vi "SRDG535.evt Call Set Trigger.vi"(0 "i ref in":refnum<vi>, 2 "Generator Instance":string="N/A", 3 "Trigger Settings":T1={"trigger"=0, "Impedance"=FALSE, "Slope"=FALSE, "burst count"=2, "external level (V)"=0.0, "Internal/Burst Rate (Hz)"=0.001, "Burst Period"=4} {"Burst Period" min=4 max=32766; "Internal/Burst Rate (Hz)" min=0.001 max=1000000.0 format="%.3f"; "external level (V)" min=-2.56 max=2.56 format="%.2f"; "burst count" min=2 max=32766; "trigger" scale=0.0..4.0}, 5 "error IO":errorcluster) -> (14 "i ref out":refnum<vi>, 19 "error out":errorcluster)   [LabVIEW 2014, in "SRDG535.lvlib"]
doc: "This VI sends a simple event call."
uses:
  SRDG535.lvlib
  SRDG535.Trigger.ctl
  CSCore/CSSystem/CoreLib/CoreLib.double 2 byte array.vi
  CSCore/CSSystem/CoreLib/CoreLib.int 2 byte array.vi
  CSCore/CSSystem/CoreLib/CoreLib.short 2 byte array.vi
  CSCore/CSSystem/CoreLib/CoreLib.lvlib
  CSCore/BaseProcess/BaseProcess.lvlib
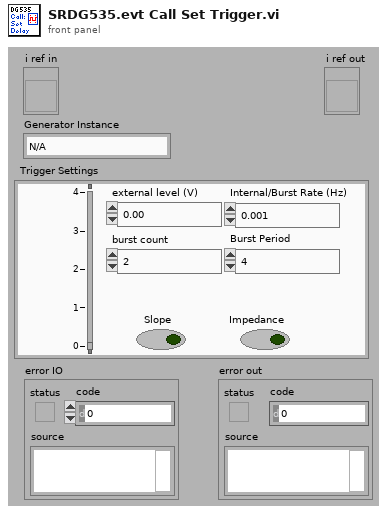
[diagram p1: front panel]
types:
  T1 = typedef "SRDG535.lvlib/SRDG535.Trigger.ctl" = cluster{"trigger":u32, "Impedance":bool, "Slope":bool, "burst count":i32, "external level (V)":sgl, "Internal/Burst Rate (Hz)":dbl, "Burst Period":i32}
  T2 = typedef "CoreDefs.rawDataType.ctl" = i8[]
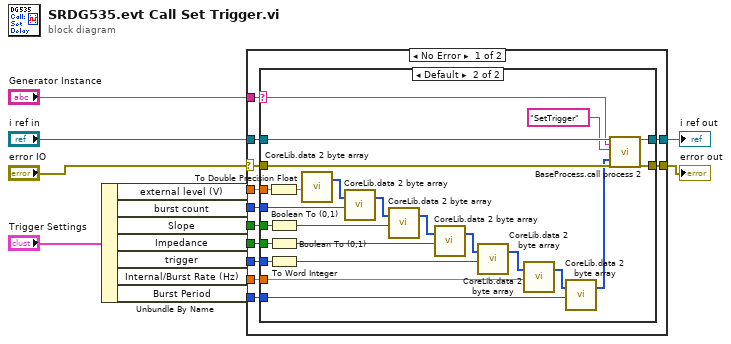
[diagram p0: block diagram]
diagram:
  n1 = Unbundle By Name("Trigger Settings") -> ("external level (V)"=w7:sgl, "burst count"=w6:i32, "Slope"=w5:bool, "Impedance"=w4:bool, "trigger"=w3:u32, "Internal/Burst Rate (Hz)"=w2:dbl, "Burst Period"=w1:i32)
  n2 = case shown="No Error" "error IO" {
    selector: "error IO" -> [w25 w52]
    tunnel: "Generator Instance" -> [w14 _]
    tunnel: [w24 w52] -> w13
    tunnel: [w22 w53] -> w12
    tunnel: w1 -> [w15 _]
    tunnel: w2 -> [w16 _]
    tunnel: w3 -> [w17 _]
    tunnel: w4 -> [w18 _]
    tunnel: w5 -> [w19 _]
    tunnel: w6 -> [w20 _]
    tunnel: w7 -> [w21 _]
    tunnel: "i ref in" -> [w23 w53]
    frame No Error {
      n3 = case shown="Default" w14 {
        selector: w14 -> [_ w32]
        tunnel: w25 -> [w26 w51]
        tunnel: [w26 w50] -> w24
        tunnel: w23 -> [w27 w49]
        tunnel: [w27 w48] -> w22
        tunnel: w21 -> [_ w41]
        tunnel: w20 -> [_ w30]
        tunnel: w19 -> [_ w40]
        tunnel: w18 -> [_ w39]
        tunnel: w17 -> [_ w29]
        tunnel: w16 -> [_ w34]
        tunnel: w15 -> [_ w33]
        frame "", "N/A" {
        }
        frame Default {
          n4 = To Double Precision Float(number=w41) -> (double precision float=w38:dbl)
          n5 = Boolean To (0,1)(Boolean=w40) -> (0, 1=w37:i16)
          n6 = Boolean To (0,1)(Boolean=w39) -> (0, 1=w36:i16)
          n7 = To Word Integer(number=w29) -> (16bit integer=w28:i16)
          n8 = call-poly "CoreLib.data 2 byte array.vi"("f64"=w38) -> ("byteArray out"=w44:T2)  [unwired: 18 in]
          n9 = call-poly "CoreLib.data 2 byte array.vi"("byteArray"=w44, "i32"=w30) -> ("byteArray out"=w43:T2)  [unwired: 17 in]
          n10 = call-poly "CoreLib.data 2 byte array.vi"("byteArray"=w43, "i16"=w37) -> ("byteArray out"=w42:T2)  [unwired: 17 in]
          n11 = call-poly "CoreLib.data 2 byte array.vi"("byteArray"=w42, "i16"=w36) -> ("byteArray out"=w35:T2)  [unwired: 17 in]
          n12 = call-poly "CoreLib.data 2 byte array.vi"("byteArray"=w35, "i16"=w28) -> ("byteArray out"=w46:T2)  [unwired: 17 in]
          n13 = call-poly "CoreLib.data 2 byte array.vi"("byteArray"=w46, "f64"=w34) -> ("byteArray out"=w45:T2)  [unwired: 17 in]
          n14 = call-poly "CoreLib.data 2 byte array.vi"("byteArray"=w45, "i32"=w33) -> ("byteArray out"=w31:T2)  [unwired: 17 in]
          n15 = call "BaseProcess.call process 2.vi"("i ref in"=w49, "Object"=w32, "Selector"="SetTrigger", "Data"=w31, "error in (no error)"=w51) -> ("i ref out"=w48:refnum<vi>, "error out"=w50:errorcluster)  [unwired: 13 in]
        }
      }
    }
    frame Error {
    }
  }
  "error out" <- w13
  "i ref out" <- w12
